vi "RichToFlatnixnet_grpc_ConvertTimestamp1nsTo100nsResponse.vi"(5 "OutputClusterType":T1, 11 "InputCluster":T2) -> (3 "OutputCluster":T1)   [LabVIEW 2025, in "xnet-grpc_client.lvlib"]
uses:
  nixnet_grpc_ConvertTimestamp1nsTo100nsResponse.ctl
  nixnet_grpc_ConvertTimestamp1nsTo100nsResponse_Flat.ctl
  xnet-grpc_client.lvlib
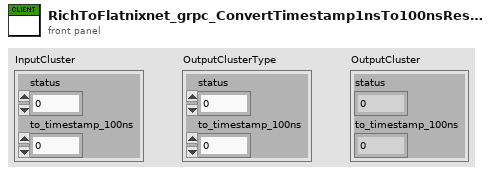
[diagram p1: front panel]
types:
  T1 = typedef "xnet-grpc_client.lvlib/nixnet_grpc_ConvertTimestamp1nsTo100nsResponse_Flat.ctl" = cluster{"status":i32, "to_timestamp_100ns":u64}
  T2 = typedef "xnet-grpc_client.lvlib/nixnet_grpc_ConvertTimestamp1nsTo100nsResponse.ctl" = cluster{"status":i32, "to_timestamp_100ns":u64}
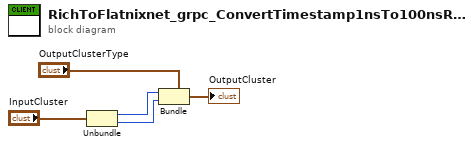
[diagram p0: block diagram]
diagram:
  n1 = Unbundle "Unbundle"("InputCluster") -> ("status"=w2:i32, "to_timestamp_100ns"=w1:u64)
  n2 = Bundle "Bundle"(cluster="OutputClusterType", "status"=w2, "to_timestamp_100ns"=w1) -> (→"OutputCluster":T1)
